vi "MGI Average (DBL[]).vi"(0 "Double[]":dbl[](array[numeric]), 1 "Ignore NaN? (F)":bool) -> (2 "Average":dbl)   [LabVIEW 2020]
doc: "This VI computes and returns the average value of the given array of doubles.\n\nAuthored by Shawn D. Walpole\nsupport@mooregoodideas.com\nwww.mooregoodideas.com\n\nCopyright (c) 2010, Moore Good Ideas, Inc.\n\nAll rights reserved.\n\nRedistribution and use in source and binary forms, with or without modification, are permitted provided that the following conditions are met:\n\n * Redistributions of source code must retain the above copyright notice, this list of conditions and the following disclaimer.\n * Redistributions in binary form must reproduce the above copyright notice, this list of conditions and the following disclaimer in the documentation and/or other materials provided with the distribution.\n * Neither the name of Moore Good Ideas, Inc. nor the names of its contributors may be used to endorse or promote products derived from this software without specific prior written permission.\n\nTHIS SOFTWARE IS PROVIDED BY THE COPYRIGHT HOLDERS AND CONTRIBUTORS \"AS IS\" AND ANY EXPRESS OR IMPLIED WARRANTIES, INCLUDING, BUT NOT LIMITED TO, THE IMPLIED WARRANTIES OF MERCHANTABILITY AND FITNESS FOR A PARTICULAR PURPOSE ARE DISCLAIMED. IN NO EVENT SHALL THE COPYRIGHT OWNER OR CONTRIBUTORS BE LIABLE FOR ANY DIRECT, INDIRECT, INCIDENTAL, SPECIAL, EXEMPLARY, OR CONSEQUENTIAL DAMAGES (INCLUDING, BUT NOT LIMITED TO, PROCUREMENT OF SUBSTITUTE GOODS OR SERVICES; LOSS OF USE, DATA, OR PROFITS; OR BUSINESS INTERRUPTION) HOWEVER CAUSED AND ON ANY THEORY OF LIABILITY, WHETHER IN CONTRACT, STRICT LIABILITY, OR TORT (INCLUDING NEGLIGENCE OR OTHERWISE) ARISING IN ANY WAY OUT OF THE USE OF THIS SOFTWARE, EVEN IF ADVISED OF THE POSSIBILITY OF SUCH DAMAGE."
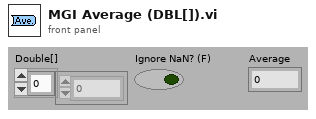
[diagram p1: front panel]
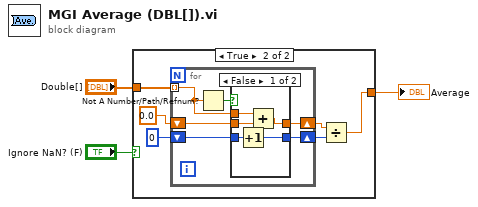
[diagram p0: block diagram]
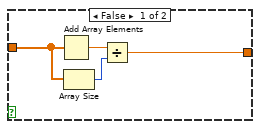
[diagram p2: hidden frame]
diagram:
  n1 = case shown="True" "Ignore NaN? (F)" {
    tunnel: "Double[]" -> [w5 w11]
    tunnel: [w4 w8] -> w2
    frame False {
      n2 = Add Array Elements(numeric array=w5) -> (sum=w7:dbl)
      n3 = Array Size(array=w5) -> (size(s)=w6:i32)
      n4 = Divide(x=w7, y=w6) -> (x/y=w4:dbl)
    }
    frame True {
      n5 = for {
        shift-right: [w14] -> w10
        shift-left: 0.0 -> [w16]
        shift-right: [w17] -> w9
        shift-left: 0 -> [w18]
        tunnel: w11 -> [w15] mode=indexing
        n6 = Not A Number/Path/Refnum?(number/path/refnum=w15) -> (NaN/Path/Refnum?=w19:bool)
        n7 = case shown="False" w19 {
          tunnel: w18 -> [w24 w25]
          tunnel: [w23 w25] -> w17
          tunnel: w16 -> [w22 w26]
          tunnel: w15 -> [w21 _]
          tunnel: [w20 w26] -> w14
          frame False {
            n8 = Increment(x=w24) -> (x+1=w23:i32)
            n9 = Add(x=w21, y=w22) -> (x+y=w20:dbl)
          }
          frame True {
          }
        }
      }
      n10 = Divide(x=w10, y=w9) -> (x/y=w8:dbl)
    }
  }
  "Average" <- w2
